vi "perform_instruction.vi"(7 "Time Since Last Instruction":dbl, 8 "error in (no error)":errorcluster, 9 "Car.lvclass":refnum<class "Car.lvclass">, 10 "Robot Properties":T1, 11 "Instruction.lvclass":refnum<class "Instruction.lvclass">) -> (0 "error out":errorcluster, 1 "Car.lvclass 2":refnum<class "Car.lvclass">, 2 "Robot Properties 2":T1, 3 "Instruction.lvclass 2":refnum<class "Instruction.lvclass">)   [LabVIEW 2015]
uses:
  class/Instruction.lvclass
  Robot.ctl
  class/Car.lvclass
  class/MovementInstruction.lvclass
  class/StopInstruction.lvclass
  class/TurnInstruction.lvclass
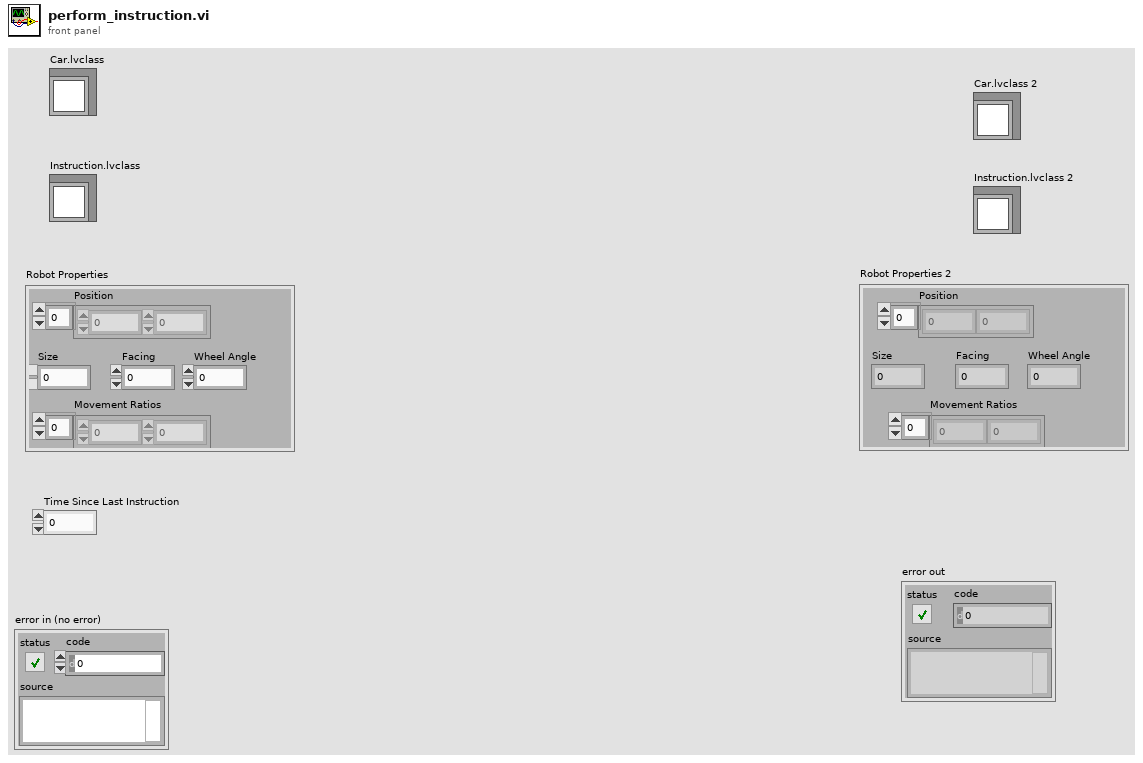
[diagram p1: front panel]
types:
  T1 = typedef "Robot.ctl" = cluster{"Position":dbl[], "Size":dbl, "Facing":dbl, "Movement Ratios":dbl[], "Wheel Angle":dbl}
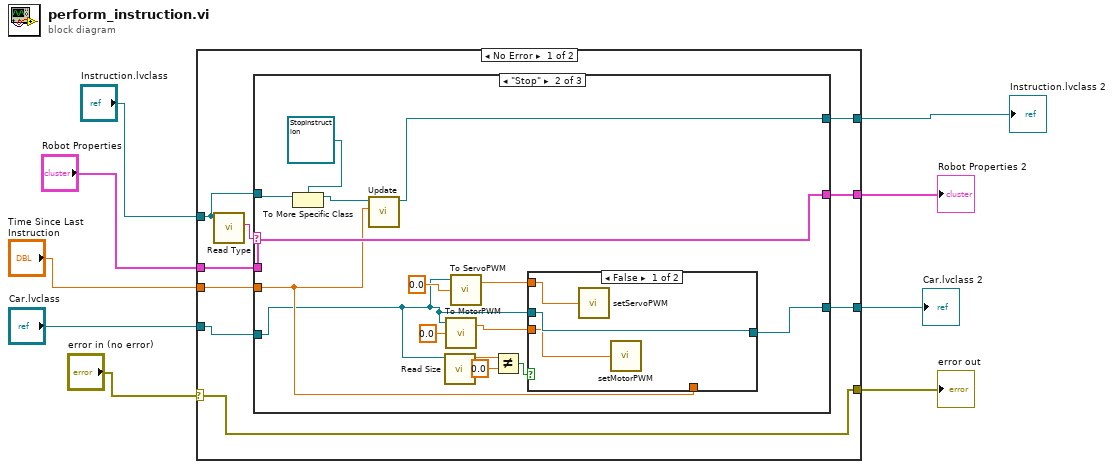
[diagram p0: block diagram]
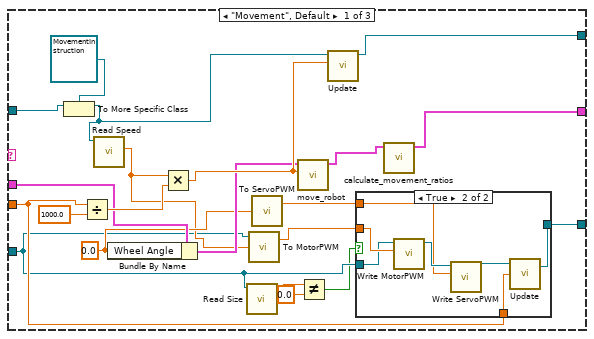
[diagram p2: hidden frame]
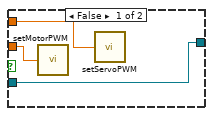
[diagram p3: hidden frame]
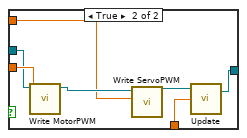
[diagram p4: hidden frame]
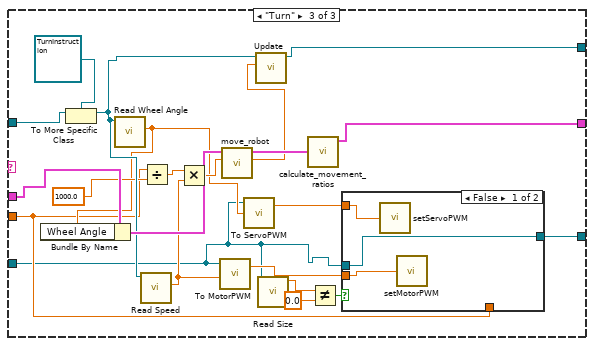
[diagram p5: hidden frame]
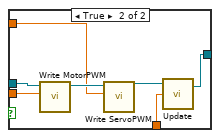
[diagram p6: hidden frame]
diagram:
  n1 = case shown="No Error" "error in (no error)" {
    selector: "error in (no error)" -> [w18 w110]
    tunnel: [w18 w110] -> w8
    tunnel: "Instruction.lvclass" -> [w16 w109]
    tunnel: "Time Since Last Instruction" -> [w15 _]
    tunnel: "Robot Properties" -> [w14 w108]
    tunnel: [w13 w108] -> w4
    tunnel: [w12 w109] -> w3
    tunnel: [w10 w107] -> w2
    tunnel: "Car.lvclass" -> [w11 w107]
    frame No Error {
      n2 = call-dynamic "Read Type.vi"("Instruction in"=w16) -> ("Type"=w17:string)  [unwired: 8 in, 2 out]
      n3 = case shown="\"Stop\"" w17 {
        tunnel: w16 -> [w38 w63 w96]
        tunnel: w15 -> [w26 w57 w80]
        tunnel: w14 -> [w30 w60 w93]
        tunnel: [w31 w60 w94] -> w13
        tunnel: [w33 w61 w90] -> w12
        tunnel: w11 -> [w22 w53 w78]
        tunnel: [w27 w54 w79] -> w10
        frame "Movement", Default {
          w25 = 0.0 ("Wheel Angle")
          n4 = To More Specific Class(target class=refnum<class "MovementInstruction.lvclass"> refnum ("MovementInstruction.lvclass"), reference=w38) -> (specific class reference=w35:refnum<class "MovementInstruction.lvclass">)  [unwired: 1 in, 1 out]
          n5 = Divide(x=w26, y=1000.0) -> (x/y=w36:dbl)
          n6 = call-dynamic "Read Speed.vi"("MovementInstruction in"=w35) -> ("Speed"=w24:dbl)  [unwired: 8 in, 2 out]
          n7 = Bundle By Name(cluster=w30, "Wheel Angle"=w25) -> (w29:T1)
          n8 = Multiply(x=w24, y=w36) -> (x*y=w34:dbl)
          n9 = call "Read Size.vi"("Car.lvclass"=w22) -> ("Size"=w21:dbl)  [unwired: 9 in, 1 out]
          n10 = call "To MotorPWM.vi"("Speed"=w24, "Car.lvclass"=w22) -> ("MotorPWM"=w23:dbl)  [unwired: 1 in, 1 out]
          n11 = call "To ServoPWM.vi"("Wheel Angle"=w25) -> ("ServoPWM"=w28:dbl)  [unwired: 2 in, 1 out]
          n12 = call "move_robot.vi"("Distance Moved"=w34, "Robot Properties"=w29) -> ("Robot Properties Out"=w32:T1)  [unwired: 8 in, 1 out]
          n13 = Not Equal?(x=w21, y=0.0) -> (x != y?=w19:bool)
          n14 = call "Update.vi"("Distance Travelled"=w34, "MovementInstruction in"=w35) -> ("MovementInstruction out"=w33:refnum<class "MovementInstruction.lvclass">)  [unwired: 8 in, 1 out]
          n15 = case shown="True" w19 {
            tunnel: w28 -> [w40 w48]
            tunnel: [w42 w46] -> w27
            tunnel: w26 -> [_ w45]
            tunnel: w23 -> [w41 w44]
            tunnel: w22 -> [w42 w43]
            frame False {
              n16 = call "setMotorPWM.vi"("Numeric"=w41) -> ()
              n17 = call "setServoPWM.vi"("Servo PWM"=w40) -> ()
            }
            frame True {
              n18 = call "Write MotorPWM.vi"("MotorPWM"=w44, "Car.lvclass"=w43) -> ("Car.lvclass 2"=w49:refnum<class "Car.lvclass">)  [unwired: 8 in, 1 out]
              n19 = call "Write ServoPWM.vi"("ServoPWM"=w48, "Car.lvclass"=w49) -> ("Car.lvclass 2"=w47:refnum<class "Car.lvclass">)  [unwired: 8 in, 1 out]
              n20 = call "Update.vi"("Time Since Last Update"=w45, "Car.lvclass"=w47) -> ("Car.lvclass 2"=w46:refnum<class "Car.lvclass">)  [unwired: 1 in, 1 out]
            }
          }
          n21 = call "calculate_movement_ratios.vi"("Robot Properties"=w32) -> ("Robot Properties"=w31:T1)  [unwired: 10 in]
        }
        frame "Stop" {
          n22 = To More Specific Class(target class=refnum<class "StopInstruction.lvclass"> refnum ("StopInstruction.lvclass"), reference=w63) -> (specific class reference=w62:refnum<class "StopInstruction.lvclass">)  [unwired: 1 in, 1 out]
          n23 = call-dynamic "Update.vi"("Time Waited"=w57, "StopInstruction in"=w62) -> ("StopInstruction out"=w61:refnum<class "StopInstruction.lvclass">)  [unwired: 8 in, 1 out]
          n24 = call "Read Size.vi"("Car.lvclass"=w53) -> ("Size"=w52:dbl)  [unwired: 9 in, 1 out]
          n25 = call "To MotorPWM.vi"("Speed"=0.0, "Car.lvclass"=w53) -> ("MotorPWM"=w59:dbl)  [unwired: 1 in, 1 out]
          n26 = call "To ServoPWM.vi"("Wheel Angle"=0.0, "Car.lvclass 2"=w53) -> ("ServoPWM"=w58:dbl)  [unwired: 1 in, 1 out]
          n27 = Not Equal?(x=w52, y=0.0) -> (x != y?=w50:bool)
          n28 = case shown="False" w50 {
            tunnel: w59 -> [w66 w74]
            tunnel: w58 -> [w65 w72]
            tunnel: w57 -> [_ w70]
            tunnel: [w67 w69] -> w54
            tunnel: w53 -> [w67 w68]
            frame False {
              n29 = call "setServoPWM.vi"("Servo PWM"=w65) -> ()
              n30 = call "setMotorPWM.vi"("Numeric"=w66) -> ()
            }
            frame True {
              n31 = call "Write MotorPWM.vi"("MotorPWM"=w74, "Car.lvclass"=w68) -> ("Car.lvclass 2"=w73:refnum<class "Car.lvclass">)  [unwired: 8 in, 1 out]
              n32 = call "Write ServoPWM.vi"("ServoPWM"=w72, "Car.lvclass"=w73) -> ("Car.lvclass 2"=w71:refnum<class "Car.lvclass">)  [unwired: 8 in, 1 out]
              n33 = call "Update.vi"("Time Since Last Update"=w70, "Car.lvclass"=w71) -> ("Car.lvclass 2"=w69:refnum<class "Car.lvclass">)  [unwired: 1 in, 1 out]
            }
          }
        }
        frame "Turn" {
          n34 = To More Specific Class(target class=refnum<class "TurnInstruction.lvclass"> refnum ("TurnInstruction.lvclass"), reference=w96) -> (specific class reference=w88:refnum<class "TurnInstruction.lvclass">)  [unwired: 1 in, 1 out]
          n35 = call-dynamic "Read Wheel Angle.vi"("TurnInstruction in"=w88) -> ("Wheel Angle"=w82:dbl)  [unwired: 8 in, 2 out]
          n36 = Bundle By Name(cluster=w93, "Wheel Angle"=w82) -> (w92:T1)
          n37 = call-dynamic "Read Speed.vi"("TurnInstruction in"=w88) -> ("Speed"=w84:dbl)  [unwired: 8 in, 2 out]
          n38 = Divide(x=w80, y=1000.0) -> (x/y=w85:dbl)
          n39 = Multiply(x=w85, y=w84) -> (x*y=w86:dbl)
          n40 = call "To MotorPWM.vi"("Speed"=w84, "Car.lvclass"=w78) -> ("MotorPWM"=w83:dbl)  [unwired: 1 in, 1 out]
          n41 = call "move_robot.vi"("Distance Moved"=w86, "Robot Properties"=w92) -> ("Angle Turned"=w91:dbl, "Robot Properties Out"=w95:T1)  [unwired: 8 in]
          n42 = call "To ServoPWM.vi"("Wheel Angle"=w82, "Car.lvclass 2"=w78) -> ("ServoPWM"=w81:dbl)  [unwired: 1 in, 1 out]
          n43 = call "Update.vi"("Angle Turned"=w91, "TurnInstruction.lvclass"=w88) -> ("TurnInstruction.lvclass 2"=w90:refnum<class "TurnInstruction.lvclass">)  [unwired: 8 in, 1 out]
          n44 = call "Read Size.vi"("Car.lvclass"=w78) -> ("Size"=w76:dbl)  [unwired: 9 in, 1 out]
          n45 = call "calculate_movement_ratios.vi"("Robot Properties"=w95) -> ("Robot Properties"=w94:T1)  [unwired: 10 in]
          n46 = Not Equal?(x=w76, y=0.0) -> (x != y?=w77:bool)
          n47 = case shown="False" w77 {
            tunnel: w83 -> [w97 w106]
            tunnel: w81 -> [w98 w104]
            tunnel: w80 -> [_ w102]
            tunnel: [w99 w101] -> w79
            tunnel: w78 -> [w99 w100]
            frame False {
              n48 = call "setServoPWM.vi"("Servo PWM"=w98) -> ()
              n49 = call "setMotorPWM.vi"("Numeric"=w97) -> ()
            }
            frame True {
              n50 = call "Write MotorPWM.vi"("MotorPWM"=w106, "Car.lvclass"=w100) -> ("Car.lvclass 2"=w105:refnum<class "Car.lvclass">)  [unwired: 8 in, 1 out]
              n51 = call "Write ServoPWM.vi"("ServoPWM"=w104, "Car.lvclass"=w105) -> ("Car.lvclass 2"=w103:refnum<class "Car.lvclass">)  [unwired: 8 in, 1 out]
              n52 = call "Update.vi"("Time Since Last Update"=w102, "Car.lvclass"=w103) -> ("Car.lvclass 2"=w101:refnum<class "Car.lvclass">)  [unwired: 1 in, 1 out]
            }
          }
        }
      }
    }
    frame Error {
    }
  }
  "Instruction.lvclass 2" <- w3
  "Robot Properties 2" <- w4
  "error out" <- w8
  "Car.lvclass 2" <- w2
